vi "SubVI_Example_GetPixelClockList.vi"(8 "error in (no error)":errorcluster, 11 ".NET (Reference)":refnum<k24>) -> (0 "error out":errorcluster, 2 "Current":i32, 3 "List":i32[](array[numeric]))   [LabVIEW 2017]
uses:
  C:/Users/George Sirinakis/Desktop/Microscope Control/Device Library/Cameras/IDS/IDS LabView Examples/LabVIEW/ueye.NET/uEyeDotNet.dll
  uEyeDotNet.dll
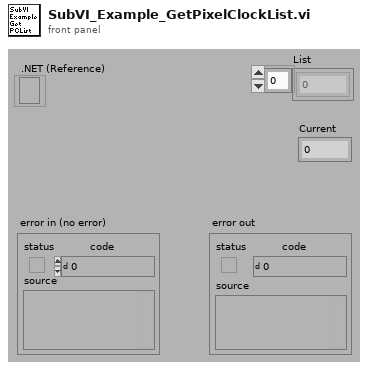
[diagram p1: front panel]
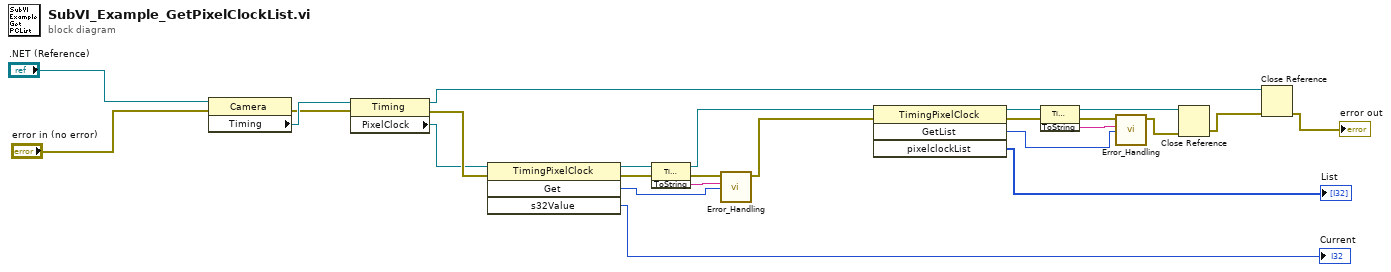
[diagram p0: block diagram]
diagram:
  n1 = property class="Camera"(reference=".NET (Reference)", error in="error in (no error)") -> (error out=w23:errorcluster, "Timing"=w24:refnum<k24>)  [unwired: 1 out]
  n2 = property class="Timing"(reference=w24, error in=w23) -> (reference out=w22:refnum<k24>, error out=w12:errorcluster, "PixelClock"=w11:refnum<k24>)
  n3 = invoke class="TimingPixelClock" method="Get"(reference=w11, error in=w12) -> (reference out=w10:refnum<k24>, error out=w9:errorcluster, "Get"=w6:i32, "s32Value"=→"Current":i32)  [unwired: 2 in]
  n4 = invoke class="TimingPixelClock" method="ToString"(reference=w10, error in=w9) -> (reference out=w3:refnum<k24>, error out=w8:errorcluster, "ToString"=w7:string)  [unwired: 1 in]
  n5 = call "Error_Handling.vi"("Error Code"=w6, "Error String"=w7, "Error In"=w8) -> ("Error Out"=w2:errorcluster)  [unwired: 8 in]
  n6 = invoke class="TimingPixelClock" method="GetList"(reference=w3, error in=w2) -> (reference out=w18:refnum<k24>, error out=w19:errorcluster, "GetList"=w13:i32, "pixelclockList"=→"List":i32[])  [unwired: 2 in]
  n7 = invoke class="TimingPixelClock" method="ToString"(reference=w18, error in=w19) -> (reference out=w17:refnum<k24>, error out=w16:errorcluster, "ToString"=w14:string)  [unwired: 1 in]
  n8 = call "Error_Handling.vi"("Error Code"=w13, "Error String"=w14, "Error In"=w16) -> ("Error Out"=w15:errorcluster)  [unwired: 8 in]
  n9 = Close Reference(reference=w17, error in (no error)=w15) -> (error out=w21:errorcluster)
  n10 = Close Reference(reference=w22, error in (no error)=w21) -> (error out=→"error out":errorcluster)
